vi "Button.vi"(3 "Set Mode":enum16{"Noop", "Button", "Switch"}(ring), 4 "In":bool, 5 "Name":string) -> (0 "Trailing":bool, 1 "Leading":bool, 2 "Out":bool)   [LabVIEW 2013, in "femtoRoboLib.lvlib"]
doc: "Create/update a Button. Has two modes, Button and Switch. If a Button, Out is True as long as button is held. If a Switch, pressing the button toggles Out. In both cases, Leading is True on the leading edge of a button press and Trailing is True on the trailing edge."
uses:
  femtoRoboLib.lvlib
  Button Control.ctl
panel:
  in  "Buttons":T1[](array[typedef])
  in  "Names":string[](array[string])
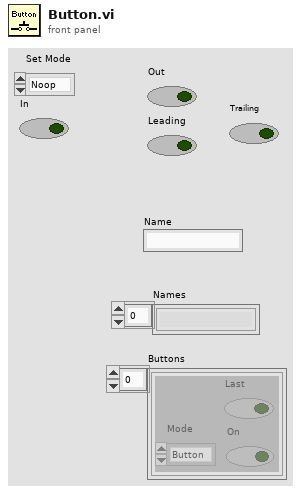
[diagram p1: front panel]
types:
  T1 = typedef "femtoRoboLib.lvlib/Button Control.ctl" = cluster{"Last":bool, "Mode":enum16{"Button", "Switch"}, "On":bool}
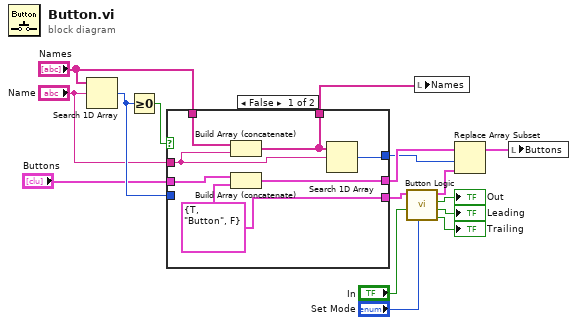
[diagram p0: block diagram]
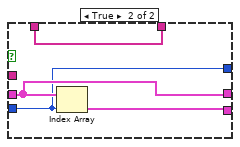
[diagram p2: hidden frame]
diagram:
  n1 = Search 1D Array(1D array="Names", element="Name") -> (index of element=w16:i32)  [unwired: 1 in]
  n2 = Greater Or Equal To 0?(x=w16) -> (x >= 0?=w14:bool)
  n3 = case shown="False" w14 {
    tunnel: w16 -> [_ w24]
    tunnel: [w17 w27] -> w7
    tunnel: "Buttons" -> [w22 w25]
    tunnel: "Names" -> [w23 w26]
    tunnel: "Name" -> [w18 _]
    tunnel: [w20 w26] -> w11
    tunnel: [w21 w25] -> w10
    tunnel: [w19 w24] -> w9
    frame False {
      w17 = T1 {"Last"=TRUE, "Mode"=enum."Button", "On"=FALSE} ("Button In")
      n4 = Build Array (concatenate)(w23, w18) -> (w20:string[])
      n5 = Build Array (concatenate)(w22, w17) -> (w21:T1[])
      n6 = Search 1D Array(1D array=w20, element=w18) -> (index of element=w19:i32)  [unwired: 1 in]
    }
    frame True {
      n7 = Index Array(array=w25, index=w24) -> (element=w27:T1)
    }
  }
  n8 = call "Button Logic.vi"("Set Mode"="Set Mode", "In"="In", "Button In"=w7) -> ("Trailing"=→"Trailing":bool, "Leading"=→"Leading":bool, "Out"=→"Out":bool, "Button Out"=w3:T1)  [unwired: 3 in]
  n9 = local write "Names"(w11) -> ()
  n10 = Replace Array Subset(array=w10, new element=w3, index=w9) -> (w8:T1[])
  n11 = local write "Buttons"(w8) -> ()
